vi "Threshold_CTAH_Inlet.vi"(6 "higher threshold":i32, 9 "BT-43":sgl, 10 "lower threshold":i32, 11 "Digital in":refnum<vi>) -> ()   [LabVIEW 2017]
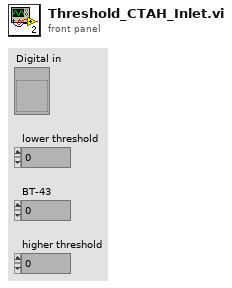
[diagram p1: front panel]
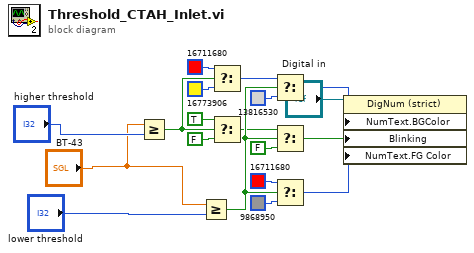
[diagram p0: block diagram]
diagram:
  n1 = Greater Or Equal?(x="BT-43", y="higher threshold") -> (x >= y?=w13:bool)
  n2 = Greater Or Equal?(x="BT-43", y="lower threshold") -> (x >= y?=w14:bool)
  n3 = Select(t=u32 16711680, s=w13, f=u32 16773906) -> (s? t:f=w4:u32)
  n4 = Select(t=TRUE ("Blinking"), s=w13, f=FALSE ("Blinking")) -> (s? t:f=w10:bool)
  n5 = Select(t=w4, s=w14, f=u32 13816530) -> (s? t:f=w18:u32)
  n6 = Select(t=w10, s=w14, f=FALSE ("Blinking")) -> (s? t:f=w17:bool)
  n7 = Select(t=u32 16711680, s=w14, f=u32 9868950) -> (s? t:f=w19:u32)
  n8 = property on="Property Node" class="DigNum (strict)"(reference="Digital in", "NumText.BGColor"=w18, "Blinking"=w17, "NumText.FG Color"=w19) -> ()  [unwired: 1 in, 2 out]
